vi "DAQmx Create Channel (AI-Acceleration-Accelerometer).vi"(0 "task in":refnum<k21>, 1 "maximum value":dbl=5.0 format="%0.2f", 2 "minimum value":dbl=-5.0 format="%0.2f", 3 "input terminal configuration":i32(ring)=-1 items=["default"=-1, "RSE"=10083, "NRSE"=10078, "Differential"=10106, "Pseudodifferential"=12529], 5 "physical channels":tag, 6 "current excitation source":i32(ring)=10200 items=["Internal"=10200, "External"=10167, "None"=10230], 7 "name to assign":string, 8 "current excitation value":dbl=0.004, 9 "units":i32(ring)=10186 items=["g"=10186, "m/s^2"=12470, "in/s^2"=12471, "From Custom Scale"=10065], 11 "error in":errorcluster, 12 "custom scale name":tag, 13 "sensitivity":dbl=1000.0, 14 "sensitivity units":i32(ring)=12509 items=["mVolts/g"=12509, "Volts/g"=12510]) -> (4 "task out":refnum<k21>, 15 "error out":errorcluster)   [LabVIEW 2011]
doc: "Creates channel(s) that use an accelerometer to measure acceleration."
uses:
  C:/Program Files/National Instruments/LabVIEW 2011/resource/objmgr/daqmx.rc
panel:
  # "input limits"
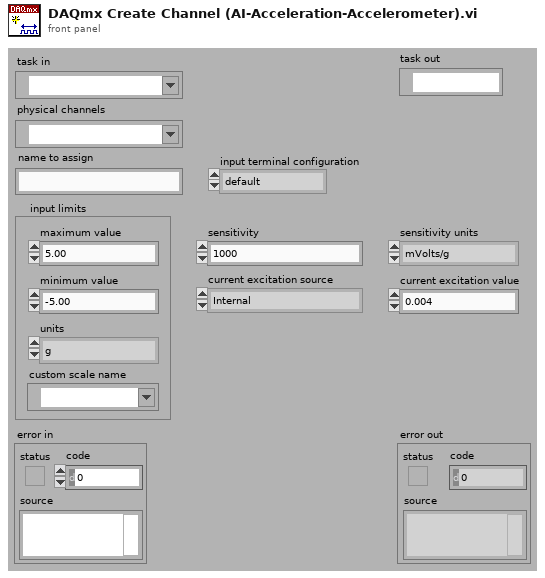
[diagram p1: front panel]
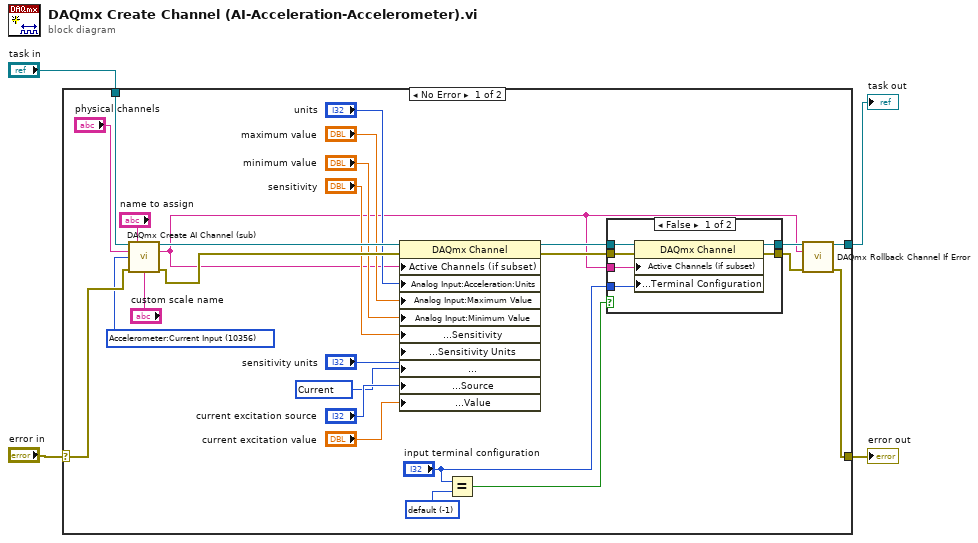
[diagram p0: block diagram]
diagram:
  n1 = case shown="No Error" "error in" {
    selector: "error in" -> [w28 w40]
    tunnel: [w20 w40] -> w2
    tunnel: "task in" -> [w29 w39]
    tunnel: [w21 w39] -> w1
    frame No Error {
      w8 = -1 items=["default"=-1, "differential"=10106, "RSE"=10083, "NRSE"=10078] ("input terminal configuration")
      w15 = 10134 items=["Voltage"=10322, "Current"=10134] ("AI.Excit.VoltageOrCurrent")
      w16 = 10356 items=["Voltage"=10322, "Current"=10134, "More:Voltage:Custom with Excitation"=10323, "More:Current:Custom with Excitation"=10136, "Frequency"=10181, "Period"=10257, "Resistance"=10278, "Temperature:Thermocouple"=10303, "Temperature:Thermistor"=10302, "Temperature:RTD"=10301, "Temperature:Built-in Sensor"=10311, "Strain Gage"=10300, "LVDT"=10352, "RVDT"=10353, "Accelerometer:Voltage Input"=10355, "Accelerometer:Current Input"=10356] ("measurement type")
      n2 = call "DAQmx Create AI Channel (sub).vi"("task in"=w29, "virtual channel name"="name to assign", "physical channel name"="physical channels", "measurement type"=w16, "error in"=w28, "custom scale"="custom scale name") -> ("task out"=w30:refnum<k21>, "channel names"=w5:string, "error out"=w25:errorcluster)  [unwired: 1 in, 6 out]
      n3 = property class="DAQmx Channel"(reference=w30, error in=w25, "Active Channels (if subset)"=w5, "Analog Input:Acceleration:Units"="units", "Analog Input:Maximum Value"="maximum value", "Analog Input:Minimum Value"="minimum value", "Analog Input:Acceleration:Accelerometer:Sensitivity"="sensitivity", "Analog Input:Acceleration:Accelerometer:Sensitivity Units"="sensitivity units", "Analog Input:General Properties:Signal Conditioning:Excitation:Advanced:Voltage or Current"=w15, "Analog Input:General Properties:Signal Conditioning:Excitation:Source"="current excitation source", "Analog Input:General Properties:Signal Conditioning:Excitation:Value"="current excitation value") -> (reference out=w12:refnum<k21>, error out=w10:errorcluster)
      n4 = Equal?(x="input terminal configuration", y=w8) -> (x = y?=w7:bool)
      n5 = case shown="False" w7 {
        tunnel: w10 -> [w36 w38]
        tunnel: [w35 w37] -> w11
        tunnel: [w34 w38] -> w9
        tunnel: "input terminal configuration" -> [w33 _]
        tunnel: w5 -> [w32 _]
        tunnel: w12 -> [w31 w37]
        frame False {
          n6 = property class="DAQmx Channel"(reference=w31, error in=w36, "Active Channels (if subset)"=w32, "Analog Input:General Properties:Input Configuration:Terminal Configuration"=w33) -> (reference out=w35:refnum<k21>, error out=w34:errorcluster)
        }
        frame True {
        }
      }
      n7 = call "DAQmx Rollback Channel If Error.vi"("task in"=w11, "channel names"=w5, "error in"=w9) -> ("task out"=w21:refnum<k21>, "error out"=w20:errorcluster)  [unwired: 11 out]
    }
    frame Error {
    }
  }
  "error out" <- w2
  "task out" <- w1
